vi "FlowFilmVariable.vi"() -> ()   [LabVIEW 2015]
panel:
  out "Flow":dbl
  out "Film Height":dbl
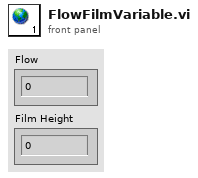
[diagram p1: front panel]
diagram:
